vi "Set Gate.vi"(9 "stepRenamed":sgl, 10 "width":sgl, 11 "delay":sgl) -> (3 "function return":u32)   [LabVIEW 2018, in "Copy of Andor SDK.lvlib"]
doc: "EXPNETTYPE unsigned int WINAPI SetGate(float delay, float width, float stepRenamed);"
uses:
  Copy of Andor SDK.lvlib
  <userlib>/Andor SDK/ATMCD32D.dll
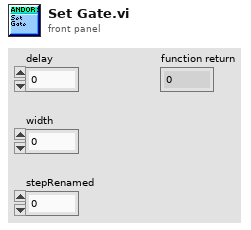
[diagram p1: front panel]
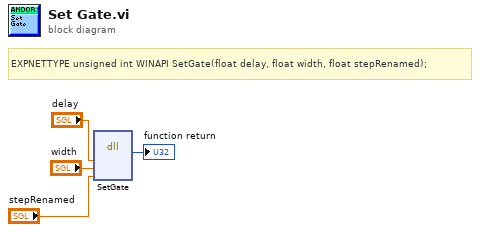
[diagram p0: block diagram]
diagram:
  # "EXPNETTYPE unsigned int WINAPI SetGate(float delay, float width, float stepRenamed);"
  n1 = dll-call lib="C:/Program Files (x86)/National Instruments/LabVIEW 2018/user.lib/Andor SDK/ATMCD32D.*" fn="SetGate"("delay"="delay", "width"="width", "stepRenamed"="stepRenamed") -> (→"function return":u32)  [unwired: 6 in, 2 out]
